vi "RPL_GUI_no2.vi"() -> ()   [LabVIEW 2021]
uses:
  <vilib>/Utility/file.llb/Read Delimited Spreadsheet (string).vi
panel:
  in  "Connection Type":u16(ring) items=["USB", "Ethernet"]
  in  "U6 Address":string="192.168.1.199"
  out "POWER DISCONNECTED":bool
  in  "?":bool
  in  "SV6 2":bool
  in  "SV5 2":bool
  in  "SV4 2":bool
  in  "START/STOP DATA LOGGING":bool
  in  "?":bool
  in  "SV3 2":bool
  in  "SV2 2":bool
  in  "SV1 2":bool
  in  "SV0 2":bool
  out "ABORT\nACTIVATED":bool
  in  "GUITabs":T1(tab) caption="Tab Control"
  out "N2O Runtank [g/s]":i16(slide) scale=0.0..100.0
  out "Ethanol Runtank [g/s]":i16(slide) scale=0.0..35.0
  out "?":bool
  out "?":bool
  out "?":bool
  out "LabJack Supply Voltage":dbl(slide) scale=0.0..5.0
  out "Solenoid Supply Voltage":dbl(slide) scale=0.0..14.0
  out "Relay Supply Voltage":dbl(slide) scale=0.0..5.0
  out "PT3: Chamber Pressure [psig]":u16(knob) scale=0.0..500.0
  in  "Arm Button":bool
  in  "Fire Button":bool
  out "DEADMAN\nSWITCH":bool
  in  "Maintain Pressure":bool
  out "IGNITION":bool
  in  "Valve Diagnostics":bool
  in  "Dry Test-Run":bool
  out "TC1: N2O Temp [°C]":i16(slide) scale=-270.0..370.0
  out "TC2: Chamber Temp [°C]":i16(slide) scale=-270.0..1260.0
  out "PT1: N2O Pressure [psig]":u16(knob) scale=0.0..1000.0
  out "PT2: Ethenol Pressure [psig]":u16(knob) scale=0.0..1000.0
  out "?":bool
  out "?":bool
  out "LP1: Thrust Reading [N]":dbl(slide) scale=0.0..200.0
  out "?":bool
  out "?":bool
  out "?":bool
  out "?":bool
  out "?":bool
  out "?":bool
  out "?":bool
  out "?":bool
  out "?":bool
  out "?":bool
  out "?":bool
  out "?":bool
  out "?":bool
  out "?":bool
  out "?":bool
  out "?":bool
  out "?":bool
  in  "Deadman Switch Pin":u16(ring) items=["FIO0", "FIO1", "FIO2", "FIO3", "FIO4", "FIO5", "FIO6", "FIO7", "EIO0", "EIO1", "EIO2", "EIO3", "EIO4", "EIO5", "EIO6", "EIO7", "CIO0", "CIO1", "CIO2", "CIO3", "MIO0", "MIO1", "MIO2"]
  in  "Solenoid Supply Pin":u16=5
  in  "LabJack Supply Pin":u16=7
  in  "Relay Supply Pin":u16=9
  in  "S: NO/NC 7":bool=TRUE
  in  "SV0 Pin":u16(ring)=8 items=["FIO0", "FIO1", "FIO2", "FIO3", "FIO4", "FIO5", "FIO6", "FIO7", "EIO0", "EIO1", "EIO2", "EIO3", "EIO4", "EIO5", "EIO6", "EIO7", "CIO0", "CIO1", "CIO2", "CIO3", "MIO0", "MIO1", "MIO2"]
  in  "SV1 3":u16(ring)=9 items=["FIO0", "FIO1", "FIO2", "FIO3", "FIO4", "FIO5", "FIO6", "FIO7", "EIO0", "EIO1", "EIO2", "EIO3", "EIO4", "EIO5", "EIO6", "EIO7", "CIO0", "CIO1", "CIO2", "CIO3", "MIO0", "MIO1", "MIO2"]
  in  "SV3 Pin":u16(ring)=11 items=["FIO0", "FIO1", "FIO2", "FIO3", "FIO4", "FIO5", "FIO6", "FIO7", "EIO0", "EIO1", "EIO2", "EIO3", "EIO4", "EIO5", "EIO6", "EIO7", "CIO0", "CIO1", "CIO2", "CIO3", "MIO0", "MIO1", "MIO2"]
  in  "SV2 Pin":u16(ring)=10 items=["FIO0", "FIO1", "FIO2", "FIO3", "FIO4", "FIO5", "FIO6", "FIO7", "EIO0", "EIO1", "EIO2", "EIO3", "EIO4", "EIO5", "EIO6", "EIO7", "CIO0", "CIO1", "CIO2", "CIO3", "MIO0", "MIO1", "MIO2"]
  in  "SV6 Pin":u16(ring)=14 items=["FIO0", "FIO1", "FIO2", "FIO3", "FIO4", "FIO5", "FIO6", "FIO7", "EIO0", "EIO1", "EIO2", "EIO3", "EIO4", "EIO5", "EIO6", "EIO7", "CIO0", "CIO1", "CIO2", "CIO3", "MIO0", "MIO1", "MIO2"]
  in  "SV5 Pin":u16(ring)=13 items=["FIO0", "FIO1", "FIO2", "FIO3", "FIO4", "FIO5", "FIO6", "FIO7", "EIO0", "EIO1", "EIO2", "EIO3", "EIO4", "EIO5", "EIO6", "EIO7", "CIO0", "CIO1", "CIO2", "CIO3", "MIO0", "MIO1", "MIO2"]
  in  "SV4 Pin":u16(ring)=12 items=["FIO0", "FIO1", "FIO2", "FIO3", "FIO4", "FIO5", "FIO6", "FIO7", "EIO0", "EIO1", "EIO2", "EIO3", "EIO4", "EIO5", "EIO6", "EIO7", "CIO0", "CIO1", "CIO2", "CIO3", "MIO0", "MIO1", "MIO2"]
  in  "S: NO/NC 6":bool=TRUE
  in  "S: NO/NC 5":bool=TRUE
  in  "S: NO/NC 4":bool=TRUE
  in  "S: NO/NC 3":bool=TRUE
  in  "S: NO/NC 2":bool
  in  "S: NO/NC":bool
  in  "R: NC/NO 7":bool=TRUE
  in  "R: NC/NO 6":bool=TRUE
  in  "R: NC/NO 5":bool=TRUE
  in  "R: NC/NO 4":bool=TRUE
  in  "R: NC/NO 3":bool=TRUE
  in  "R: NC/NO 2":bool=TRUE
  in  "R: NC/NO":bool=TRUE
  in  "?":bool
  in  "TC1 Type":u16(ring)=7 items=["B", "E", "J", "K", "N", "R", "S", "T"]
  in  "TC2 Type":u16(ring)=3 items=["B", "E", "J", "K", "N", "R", "S", "T"]
  in  "TC1 +Channel":u16
  in  "TC2 -Channel":u16=3
  in  "TC2 +Channel":u16=2
  in  "TC1 -Channel":u16=1
  in  "PT2 Pin":u16=6
  in  "PT1 Pin":u16=8
  in  "PT3 Pin":u16=4
  in  "LP1 Pin":u16=10
  in  "k [N/m]":dbl=2000.0
  out "?":u32[](array[numeric])
  out "?":bool[](array[boolean])
  out "?":string[](array[string])
  in  "SV0":bool
  out "?":bool[](array[boolean])
  out "?":bool[](array[boolean])
  out "?":bool[](array[boolean])
  in  "SV1":bool
  in  "SV2":bool
  in  "SV3":bool
  out "?":bool[](array[boolean])
  in  "SV4":bool
  out "?":bool[](array[boolean])
  out "?":bool[](array[boolean])
  in  "SV5":bool
  in  "SV6":bool
  in  "Procedure Name":string
  in  "P#":u32
  in  "Add Procedure":bool
  in  "Remove Procedure":bool
  in  "Row 2":u32
  out "Row":u32[](array[numeric])
  out "File Path":path[](array[path])
  # "LINE & CHAMBER STATUS"
  # "HIL TEST PARAMETERS"
  # "SYSTEM FIRE OPERATION"
  # "DIAGNOSTIC TEST-RUN"
  # "THRUST STATUS"
  # "RUNTANK FLOWRATE STATUS"
  # "SYSTEM ERROR CALLSTACK"
  # "DATA LOGGING"
  # "PRESSURE TRANSMITTER SETTINGS"
  # "THERMOCOUPLE SETTINGS"
  # "SOLENOID VALVE & RELAY SETTINGS"
  # "CALIBRATION SETTINGS"
  # "SYSTEM POWER SETTINGS"
  # "LINEAR POTENTIOMETER SETTINGS"
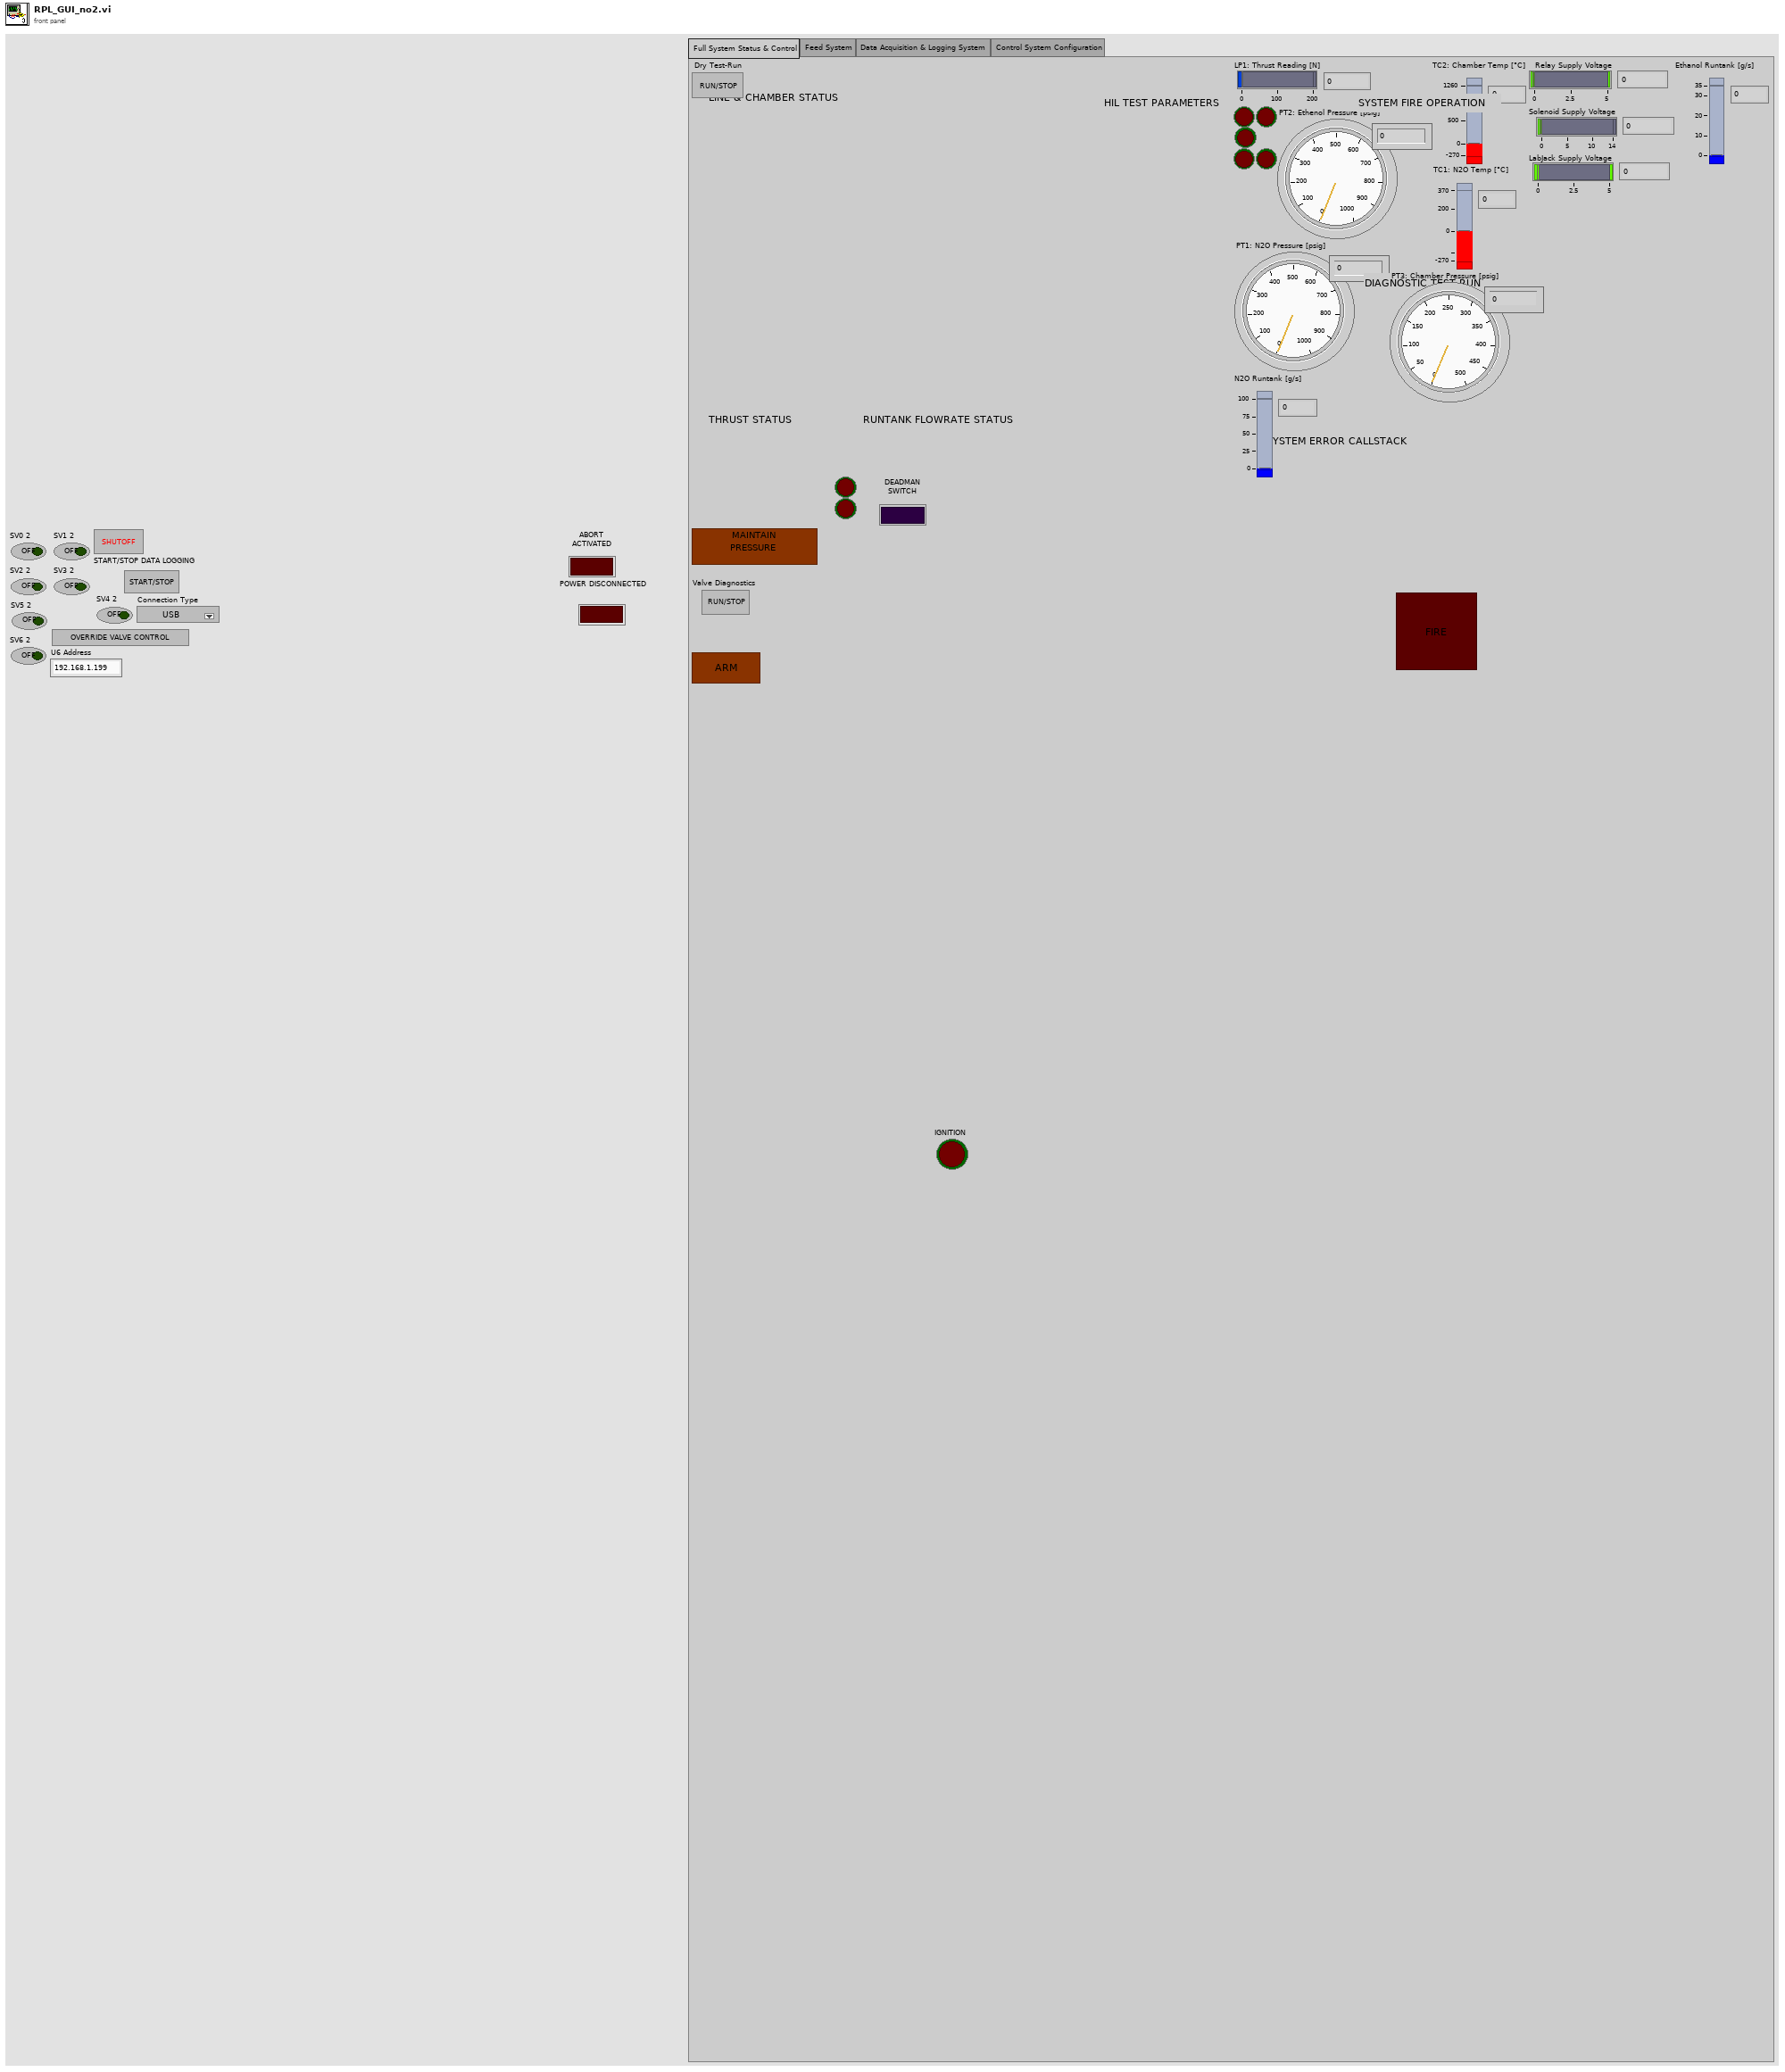
[diagram p1: front panel]
types:
  T1 = enum32{"Full System Status & Control", "Feed System", "Data Acquisition & Logging System", "Control System Configuration"}
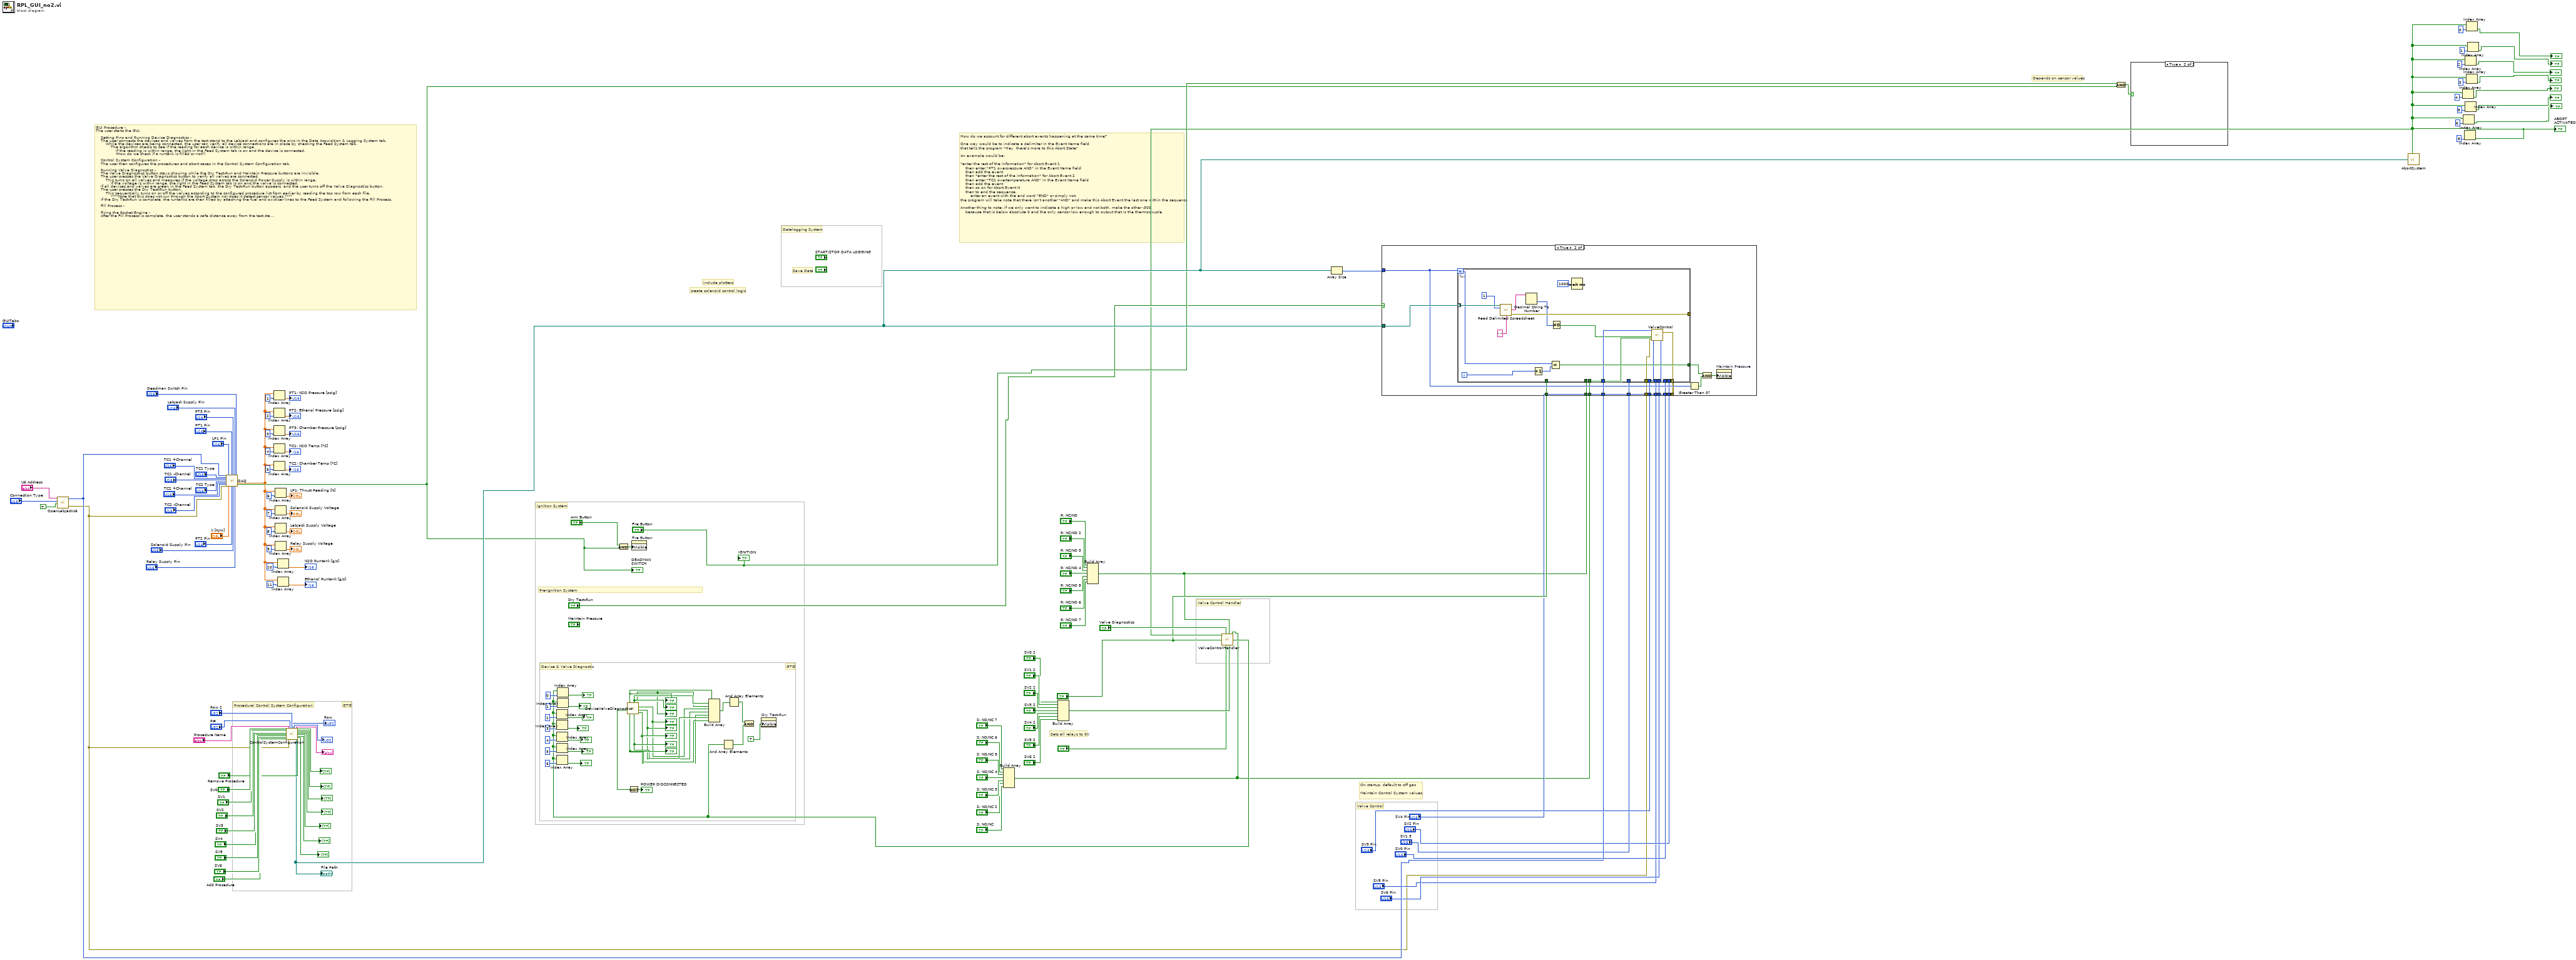
[diagram p0: block diagram]
diagram:
  # "Depends on sensor values"
  # "GTG"
  # "GTG"
  # "On startup, default to off gas\n\nMaintain Control System values."
  # "Procedural Control System Configuration"
  # "Pre-Ignition System"
  # "GUI Procedure -\nThe user starts the GUI.\n\n    Setting Pins and Running Device Diagnostics -\n    The user connects the devices and valves from the test stand to the LabJack and configures the pins in the Data Acquisition & Logging System tab.\n        While the devices are being connected, the user can verify all device connections are in place by checking the Feed System tab.\n            The algorithm checks to see if the reading for each device is within range.\n                If the reading is within range, the light in the Feed System tab is on and the device is connected.\n                (How do we check if a runtank is filled or not?)\n\n    Control System Configuration -\n    The user then configures the procedures and abort cases in the Control System Configuration tab.\n\n    Running Valve Diagnostics -\n    The Valve Diagnostics button stays showing while the Dry Test-Run and Maintain Pressure buttons are invisible.\n    The user presses the Valve Diagnostics button to verify all valves are connected.\n        This turns on all valves and measures if the voltage drop across the Solenoid Power Supply is within range.\n            If the voltage is within range, the light in the Feed System tab is on and the valve is connected.\n    If all devices and valves are green in the Feed System tab, the Dry Test-Run button appears, and the user turns off the Valve Diagnostics button.\n    The user presses the Dry Test-Run button.\n        This sequentially turns on or off the valves according to the configured procedure list from earlier by reading the top row from each file.\n            ****Note that this does not run through the Abort System nor does it detect sensor values.****\n    If the Dry Test-Run is complete, the runtanks are then filled by attaching the fuel and oxidizer lines to the Feed System and following the Fill Process.\n\n    Fill Process -\n\n    Firing the Rocket Engine -\n    After the Fill Process is complete, the user stands a safe distance away from the test stand.\n    The runtanks are massed to check if they are filled.\n        This makes the Maintain Pressure button appear and makes the Valve Diagnostics button and the Dry Test-Run button invisible and off to avoid further misclicking.\n    The user presses the Maintain Pressure button to not let the Feed System depressurize. The rocket engine is ready to fire.\n    To fire the rocket engine, the user presses the Arm button [on the count of 3] and holds down the Deadman Switch [on the count of 2].\n        This makes the Fire button appear and makes the Maintain Pressure button invisible and off to avoid further misclicking.\n        The user presses the Fire button [on the count of 1] to fire the rocket engine."
  # "Device & Valve Diagnostic"
  # "Datalogging System"
  # "Ignition System"
  # "Save Data"
  # "Sets all relays to 0V"
  # "Valve Control Handler"
  # "How do we account for different abort events happening at the same time?\n\nOne way would be to indicate a delimiter in the Event Name field\nthat tells the program \"Hey, there's more to this Abort State\"\n\nAn example would be:\n\n*enter the rest of the information* for Abort Event 1\n    then enter \"PT1 overpressure AND\" in the Event Name field\n    then add the event\n    then *enter the rest of the information* for Abort Event 2\n    then enter \"TC1 overtemperature AND\" in the Event Name field\n    then add the event\n    then so on for Abort Event N\n    then to end the sequence,\n        enter an event with the end word \"END\" or simply not,\nthe program will take note that there isn't another \"AND\" and make this Abort Event the last one within the sequence\n\nAnother thing to note: if we only want to indicate a high or low and not both, make the other -300\n    because that is below absolute 0 and the only sensor low enough to output that is the thermocouple."
  # "Valve Control"
  # "create solenoid control logic"
  # "include plotters"
  n1 = call "OpenLabJackU6.vi"("Select First Found"=TRUE, "Connection Type"="Connection Type", "U6 Address"="U6 Address") -> ("error out"=w3:errorcluster, "Handle"=w9:i32)  [unwired: 1 in, 1 out]
  n2 = call "DAQ.vi"("Handle In"=w9, "TC1 Type"="TC1 Type", "TC1 +Channel"="TC1 +Channel", "TC1 -Channel"="TC1 -Channel", "TC2 Type"="TC2 Type", "TC2 +Channel"="TC2 +Channel", "TC2 -Channel"="TC2 -Channel", "error in"=w3, "LP1 Pin"="LP1 Pin", "k [N/m]"="k [N/m]", "PT1 Pin"="PT1 Pin", "PT2 Pin"="PT2 Pin", "PT3 Pin"="PT3 Pin", "Solenoid Supply Pin"="Solenoid Supply Pin", "LabJack Supply Pin"="LabJack Supply Pin", "Relay Supply Pin"="Relay Supply Pin", "Deadman Switch Pin"="Deadman Switch Pin") -> ("Sensor Values"=w34:dbl[], "Deadman Switch"=w13:bool)  [unwired: 8 in, 1 out]
  "DEADMAN\nSWITCH" <- w13
  n3 = Index Array(array=w34, index=1) -> (element=→"PT1: N2O Pressure [psig]":dbl)
  n4 = Index Array(array=w34, index=2) -> (element=→"PT2: Ethenol Pressure [psig]":dbl)
  n5 = Index Array(array=w34, index=3) -> (element=→"PT3: Chamber Pressure [psig]":dbl)
  n6 = Index Array(array=w34, index=4) -> (element=→"TC1: N2O Temp [°C]":dbl)
  n7 = Index Array(array=w34, index=5) -> (element=→"TC2: Chamber Temp [°C]":dbl)
  n8 = Index Array(array=w34, index=6) -> (element=→"LP1: Thrust Reading [N]":dbl)
  n9 = Index Array(array=w34, index=7) -> (element=→"Solenoid Supply Voltage":dbl)
  n10 = Index Array(array=w34, index=8) -> (element=→"LabJack Supply Voltage":dbl)
  n11 = Index Array(array=w34, index=9) -> (element=→"Relay Supply Voltage":dbl)
  n12 = Index Array(array=w34, index=10) -> (element=→"N2O Runtank [g/s]":dbl)
  n13 = Index Array(array=w34, index=11) -> (element=→"Ethanol Runtank [g/s]":dbl)
  n14 = call "ControlSystemConfiguration.vi"("SV0"="SV0", "SV1"="SV1", "SV2"="SV2", "SV3"="SV3", "SV4"="SV4", "SV5"="SV5", "SV6"="SV6", "Add Procedure"="Add Procedure", "Procedure Name"="Procedure Name", "error in"=w3, "P#"="P#", "Row"="Row 2", "Remove Procedure"="Remove Procedure") -> ("Row"=→"Row":u32[], 16:→"?":u32[], 18:→"?":string[], "File Path"=w62:path[], 20:→"?":bool[], 21:→"?":bool[], 22:→"?":bool[], 23:→"?":bool[], 24:→"?":bool[], 25:→"?":bool[], 26:→"?":bool[])  [unwired: 3 in, 1 out]
  "File Path" <- w62
  n15 = And(x="Arm Button", y=w13) -> (x .and. y?=w107:bool)
  n16 = call "DeviceValveDiagnostics.vi"() -> (0:w85:bool, "Power Connected"=w75:bool, 3:w82:bool, 4:w84:bool, 5:w81:bool, 6:w83:bool, 7:w79:bool, 8:w78:bool, 9:w80:bool)  [unwired: 1 in]
  "?" <- w79
  "?" <- w78
  "?" <- w85
  "?" <- w84
  "?" <- w83
  "?" <- w80
  "?" <- w82
  "?" <- w81
  n17 = Not(x=w75) -> (.not. x?=→"POWER DISCONNECTED":bool)
  n18 = property on="Fire Button" class="Bool (strict)"("Visible"=w107) -> ()  [unwired: 2 in, 2 out]
  n19 = Build Array(w85, w84, w83, w79, w78, w80, w81, w82) -> (w77:bool[])
  n20 = And Array Elements(Boolean array=w77) -> (logical AND=w87:bool)
  n21 = property on="Dry Test-Run" class="Bool (strict)"("Visible"=TRUE) -> ()  [unwired: 2 in, 2 out]
  n22 = Build Array("S: NO/NC 7", "S: NO/NC 6", "S: NO/NC 5", "S: NO/NC 4", "S: NO/NC 3", "S: NO/NC 2", "S: NO/NC") -> (w1:bool[])
  n23 = Build Array("SV0 2", "SV1 2", "SV2 2", "SV3 2", "SV4 2", "SV5 2", "SV6 2") -> (w105:bool[])
  n24 = Build Array("R: NC/NO", "R: NC/NO 2", "R: NC/NO 3", "R: NC/NO 4", "R: NC/NO 5", "R: NC/NO 6", "R: NC/NO 7") -> (w2:bool[])
  n25 = Array Size(array=w62) -> (size(s)=w63:i32)
  n26 = case shown="True" "Dry Test-Run" {
    tunnel: w63 -> [_ w167]
    tunnel: w62 -> [_ w170]
    tunnel: "?" -> [_ w166]
    tunnel: w2 -> [_ w165]
    tunnel: w1 -> [_ w164]
    tunnel: "SV3 Pin" -> [_ w163]
    tunnel: "SV0 Pin" -> [_ w162]
    tunnel: w9 -> [_ w161]
    tunnel: "SV1 3" -> [_ w160]
    tunnel: "SV2 Pin" -> [_ w159]
    tunnel: "SV4 Pin" -> [_ w158]
    tunnel: "SV6 Pin" -> [_ w157]
    tunnel: "SV5 Pin" -> [_ w156]
    tunnel: w3 -> [_ w155]
    frame False {
    }
    frame True {
      n27 = for {
        N: w167 -> [w185]
        tunnel: w170 -> [w193] mode=indexing
        tunnel: [w190] -> _
        tunnel: [w184] -> w169
        tunnel: w166 -> [_]
        tunnel: w165 -> [w173]
        tunnel: w164 -> [w172]
        tunnel: w163 -> [w182]
        tunnel: w162 -> [w181]
        tunnel: w161 -> [w180]
        tunnel: w160 -> [w179]
        tunnel: w159 -> [w178]
        tunnel: [w177] -> w158 mode=indexing
        tunnel: w157 -> [w176]
        tunnel: w156 -> [w175]
        tunnel: w155 -> [w174]
        i -> [w186]
        n28 = call-poly <vilib>:"Read Delimited Spreadsheet.vi"("file path (dialog if empty)"=w193, "number of rows (all:-1)"=1, "delimiter (\\t)"="," ("delimiter (\\t)")) -> ("first row"=w189:string[], "error out"=w190:errorcluster)  [unwired: 7 in, 4 out]
        n29 = Decimal String To Number(string=w189) -> (number=w188:i32[])  [unwired: 2 in, 1 out]
        n30 = Increment(x=w186) -> (x+1=w187:i32)
        n31 = Equal?(x=w185, y=w187) -> (x = y?=w184:bool)
        n32 = Not Equal To 0?(x=w188) -> (x != 0?=w171:bool[])
        n33 = Wait (ms)(milliseconds to wait=u32 1000) -> ()  [unwired: 1 out]
        n34 = call "ValveControl.vi"("SV Pin"=w173, "Solenoid States"=w181, "error in"=w174, "Solenoid NC/NO"=w171, "Relay NO/NC"=w182, "Handle In"=w180) -> ("error out"=w177:errorcluster[])
      }
      n35 = Greater Than 0?(x=w167) -> (x > 0?=w168:bool)
      n36 = And(x=w169, y=w168) -> (x .and. y?=w154:bool)
      n37 = property on="Maintain Pressure" class="Bool (strict)"("Visible"=w154) -> ()  [unwired: 2 in, 2 out]
    }
  }
  n38 = And(x="Fire Button", y=w13) -> (x .and. y?=w64:bool)
  n39 = case shown="True" w64 {
    frame False {
    }
    frame True {
    }
  }
  n40 = call "AbortSystem.vi"("File Path"=w62) -> ("Abort Status"=w65:bool[])  [unwired: 3 in, 1 out]
  n41 = Index Array(array=w65, index=4) -> (element=→"?":bool)
  n42 = Index Array(array=w65, index=6) -> (element=→"?":bool)
  n43 = Index Array(array=w65, index=8) -> (element=w52:bool)
  "ABORT\nACTIVATED" <- w52
  n44 = call "ValveControlHandler.vi"("Override Control Outputs"=w105, "Solenoid NC/NO"=w1, "Relay NO/NC"=w2, "Manual Abort"="?", "Manual Override"="?", "Valve Diagnostics"="Valve Diagnostics", "Abort"=w52) -> ("Valve Diagnostics"=w88:bool[])  [unwired: 2 in, 1 out]
  n45 = Index Array(array=w88, index=2) -> (element=→"?":bool)
  n46 = Index Array(array=w88, index=6) -> (element=→"?":bool)
  n47 = Index Array(array=w88, index=3) -> (element=→"?":bool)
  n48 = Index Array(array=w88, index=4) -> (element=→"?":bool)
  n49 = Index Array(array=w88, index=5) -> (element=→"?":bool)
  n50 = Index Array(array=w88, index=1) -> (element=→"?":bool)
  n51 = Index Array(array=w88, index=0) -> (element=→"?":bool)
  n52 = And Array Elements(Boolean array=w88) -> (logical AND=w86:bool)
  n53 = And(x=w87, y=w86) -> ()  [unwired: 1 out]
  n54 = Index Array(array=w65, index=2) -> (element=→"?":bool)
  n55 = Index Array(array=w65, index=5) -> (element=→"?":bool)
  n56 = Index Array(array=w65, index=0) -> (element=→"?":bool)
  n57 = Index Array(array=w65, index=3) -> (element=→"?":bool)
  n58 = Index Array(array=w65, index=1) -> (element=→"?":bool)
  "IGNITION" <- "Fire Button"
